vi "GetDescription.vi"(7 "$Path or Item Name":string="$.description", 8 "error in (no error)":errorcluster, 11 "Value":string) -> (0 "error out":errorcluster, 2 "description":string)   [LabVIEW 2021]
uses:
  <vilib>/JDP Science/JSONtext/JSON Value Type.ctl
  2282269b-cb8c-4795-98ad-976a2d1ac491.vi
  d729b316-12a2-412a-bbdd-9e0c31f1e354.vi
  6341a016-0793-4cbb-b524-2edbfc2684ae.vi
  5cb707a2-5937-4a4f-b254-499d7469b464.vi
  5b23f87a-f59f-4698-8b46-1a7e5f62e880.vi
  <vilib>/JDP Science/JSONtext/Next JSON Value.vi
  <vilib>/JDP Science/JSONtext/String Subset.vi
  <vilib>/JDP Science/JSONtext/Parsing/Advance past next JSON Value (inlined COPY).vi
  <vilib>/JDP Science/JSONtext/Parsing/Advance past whitespace.vi
  <vilib>/JDP Science/JSONtext/Parsing/Advance past String.vi
  <vilib>/JDP Science/JSONtext/Parsing/Advance past Number.vi
  <vilib>/JDP Science/JSONtext/Parsing/Advance past Line Ending.vi
  <vilib>/JDP Science/JSONtext/Parsing/Parse Full Path or Item Name.vi
  <vilib>/JDP Science/JSONtext/Parsing/Advance past Array.vi
  <vilib>/JDP Science/JSONtext/Parsing/Advance past Object.vi
  <vilib>/JDP Science/JSONtext/support/Error Cluster From Code.vi
  <vilib>/JDP Science/JSONtext/Offset/Find Item Locations by Path.vi
  <vilib>/JDP Science/JSONtext/JSON text to Variant.vi
  <vilib>/JDP Science/JSONtext/LVClass Serializer/JSONtext LVClass Serializer.lvclass
  <vilib>/JDP Science/JSONtext/JSONtext.lvlib
panel:
  out "JSON Value Type":T1
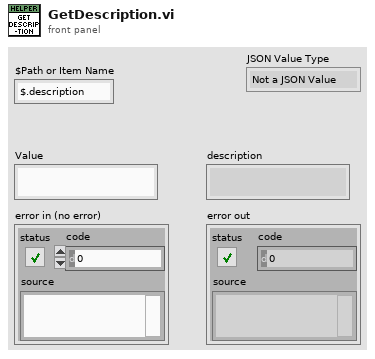
[diagram p1: front panel]
types:
  T1 = typedef "JSONtext.lvlib/JSON Value Type.ctl" = enum16{"Not a JSON Value", "JSON Object", "JSON Array", "String", "Number", "true", "false", "null"}
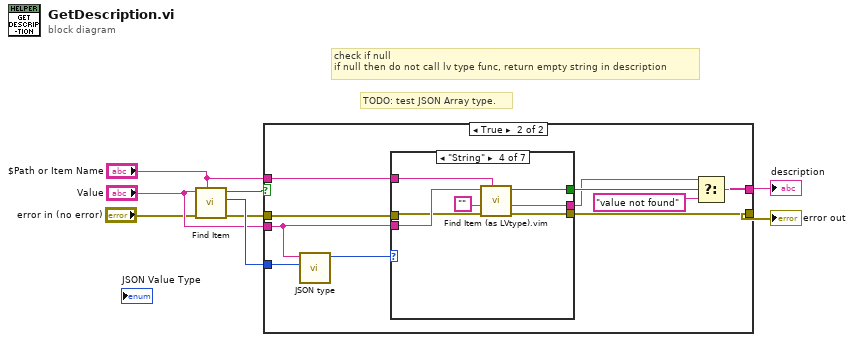
[diagram p0: block diagram]
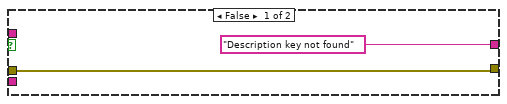
[diagram p2: hidden frame]
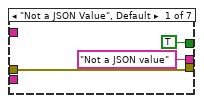
[diagram p3: hidden frame]
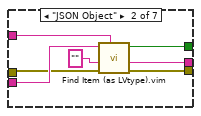
[diagram p4: hidden frame]
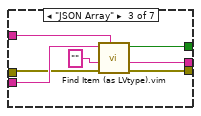
[diagram p5: hidden frame]
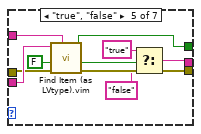
[diagram p6: hidden frame]
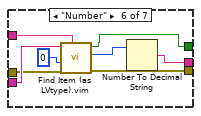
[diagram p7: hidden frame]
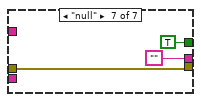
[diagram p8: hidden frame]
diagram:
  # "TODO: test JSON Array type."
  # "check if null\nif null then do not call lv type func, return empty string in description"
  n1 = call <vilib>:"Find Item.vi"("$Path or Item Name"="$Path or Item Name", "error in (no error)"="error in (no error)", "JSON"="Value") -> ("error out"=w2:errorcluster, "Item offset"=w8:i32, "Found"=w4:bool)  [unwired: 5 in, 1 out]
  n2 = case shown="True" w4 {
    tunnel: w8 -> [_ w20]
    tunnel: "Value" -> [_ w18]
    tunnel: ["Description key not found" ("Data") w12] -> w5
    tunnel: "$Path or Item Name" -> [_ w17]
    tunnel: w2 -> [w9 w16]
    tunnel: [w9 w15] -> w1
    frame False {
    }
    frame True {
      n3 = call <vilib>:"JSON type.vi"("Offset"=w20, "JSON"=w18) -> ("JSON Value Type"=w19:T1)  [unwired: 8 in, 1 out]
      n4 = case shown="\"String\"" w19 {
        tunnel: ["Not a JSON value" ("Data") w30 w37 w44 w47 w56 ""] -> w13
        tunnel: w18 -> [_ w28 w35 w43 w54 w62 _]
        tunnel: w17 -> [_ w27 w34 w42 w53 w61 _]
        tunnel: w16 -> [w23 w26 w33 w41 w52 w60 w64]
        tunnel: [w23 w25 w32 w40 w51 w59 w64] -> w15
        tunnel: [TRUE ("Found") w24 w31 w39 w45 w55 TRUE ("Found")] -> w14
        frame "Not a JSON Value", Default {
        }
        frame "JSON Object" {
          n5 = call "Find Item (as LVtype).vim"("$Path or Item Name"=w27, "error in (no error)"=w26, "Data Type and Default Value"="", "JSON"=w28) -> ("error out"=w25:errorcluster, "Data"=w30:string, "Found"=w24:bool)  [unwired: 4 in, 1 out]
        }
        frame "JSON Array" {
          n6 = call "Find Item (as LVtype).vim"("$Path or Item Name"=w34, "error in (no error)"=w33, "Data Type and Default Value"="", "JSON"=w35) -> ("error out"=w32:errorcluster, "Data"=w37:string, "Found"=w31:bool)  [unwired: 4 in, 1 out]
        }
        frame "String" {
          n7 = call "Find Item (as LVtype).vim"("$Path or Item Name"=w42, "error in (no error)"=w41, "Data Type and Default Value"="", "JSON"=w43) -> ("error out"=w40:errorcluster, "Data"=w44:string, "Found"=w39:bool)  [unwired: 4 in, 1 out]
        }
        frame "true", "false" {
          n8 = call "Find Item (as LVtype).vim"("$Path or Item Name"=w53, "error in (no error)"=w52, "Data Type and Default Value"=FALSE, "JSON"=w54) -> ("error out"=w51:errorcluster, "Data"=w49:bool, "Found"=w45:bool)  [unwired: 4 in, 1 out]
          n9 = Select(t="true", s=w49, f="false") -> (s? t:f=w47:string)
        }
        frame "Number" {
          n10 = call "Find Item (as LVtype).vim"("$Path or Item Name"=w61, "error in (no error)"=w60, "Data Type and Default Value"=0, "JSON"=w62) -> ("error out"=w59:errorcluster, "Item offset"=w57:i32, "Found"=w55:bool)  [unwired: 4 in, 1 out]
          n11 = Number To Decimal String(number=w57) -> (decimal integer string=w56:string)  [unwired: 1 in]
        }
        frame "null" {
        }
      }
      n12 = Select(t=w13, s=w14, f="value not found") -> (s? t:f=w12:string)
    }
  }
  "error out" <- w1
  "description" <- w5
